vi "array -- find monotonic segments.vi"(6 "min length of monotonic segment":i32=5, 11 "list of numbers":dbl[](array[numeric])=[1.0, 2.0, 3.0, 4.0, 4.0, 5.0, 4.0, 5.0, 3.0, 2.0, 1.0, 1.0, 2.0, 3.0, 4.0, 5.0]) -> (2 "array of monotonic segments":T1[](array[typedef]))   [LabVIEW 2015]
uses:
  array -- monotnic segment.ctl
panel:
  in  "Cluster":T1
  out "ind":i32[](array[numeric])=[1, 2, 3, 4, 4, 5, 4, 5, 3, 2, 1, 1, 2, 3, 4, 5]
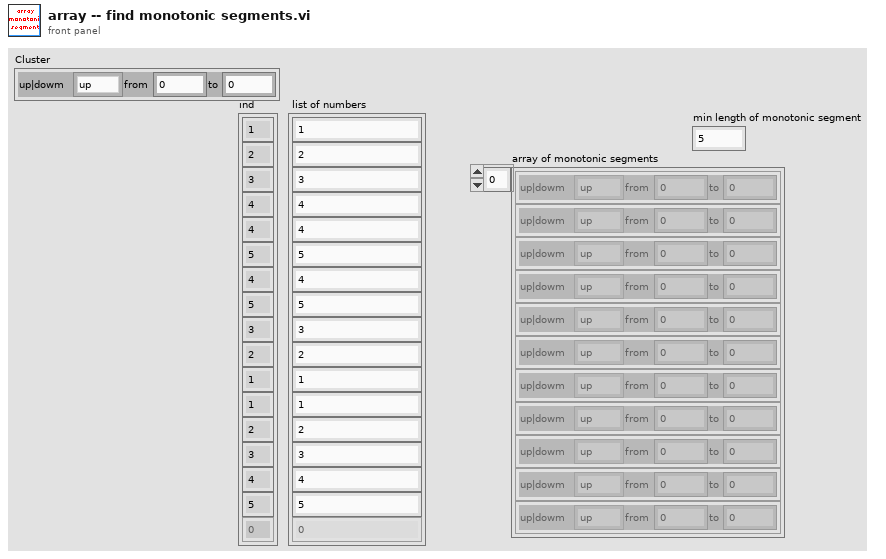
[diagram p1: front panel]
types:
  T1 = typedef "array -- monotnic segment.ctl" = cluster{"to":i32, "from":i32, "up|dowm":enum16{"up", "down"}}
  T2 = cluster{"index to":i32, "index from":i32, "up|dowm":enum16{"up", "down"}}
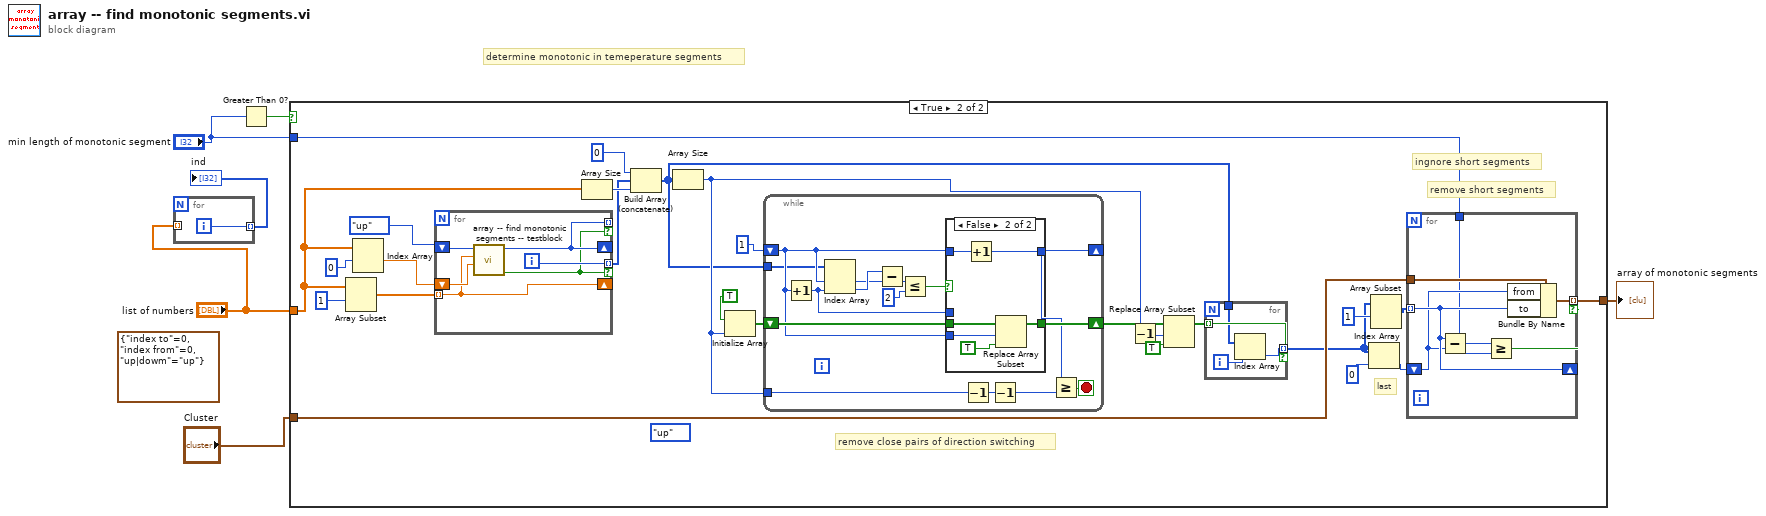
[diagram p0: block diagram]
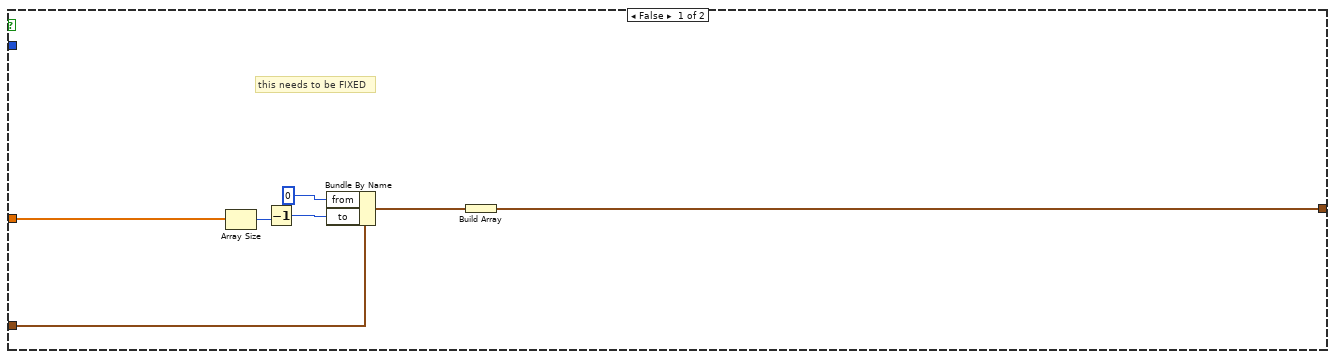
[diagram p2: hidden frame]
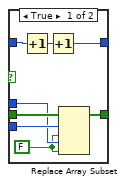
[diagram p3: hidden frame]
diagram:
  (unwired) T2 {"index to"=0, "index from"=0, "up|dowm"=enum."up"}
  # "determine monotonic in temeperature segments"
  n1 = for {
    tunnel: "list of numbers" -> [_] mode=indexing
    tunnel: [w7] -> w4 mode=indexing
    i -> [w7]
  }
  "ind" <- w4
  n2 = Greater Than 0?(x="min length of monotonic segment") -> (x > 0?=w5:bool)
  n3 = case shown="True" w5 {
    tunnel: "list of numbers" -> [w13 w28]
    tunnel: "min length of monotonic segment" -> [_ w15]
    tunnel: "Cluster" -> [w9 w33]
    tunnel: [w8 w18] -> w1
    frame False {
      # "this needs to be FIXED"
      n4 = Array Size(array=w13) -> (size(s)=w12:i32)
      n5 = Decrement(x=w12) -> (x-1=w10:i32)
      n6 = Bundle By Name(cluster=w9, "from"=0 ("index  from"), "to"=w10) -> (w14:T1)
      n7 = Build Array(w14) -> (w8:T1[])
    }
    frame True {
      (unwired) enum16{"up", "down"}."up" ("up|dowm IN")
      # "remove short segments"
      # "last"
      # "remove close pairs of direction switching"
      # "ingnore short segments"
      n8 = Array Subset(array=w28, index=1 ("dimension size")) -> (w38:dbl[])  [unwired: 1 in]
      n9 = Index Array(array=w28, index #1=0 ("dimension size")) -> (element #1=w29:dbl)  [unwired: 1 in, 1 out]
      n10 = for {
        shift-right: [w77] -> _
        shift-left: w29 -> [w78]
        tunnel: w38 -> [w77] mode=indexing
        shift-right: [w75] -> _
        shift-left: enum16{"up", "down"}."up" ("up|dowm IN") -> [w79]
        tunnel: [w76] -> w31 mode=indexing if=w74
        tunnel: [w75] -> _ mode=indexing if=w74
        i -> [w76]
        n11 = call "array -- find monotonic segments -- testblock.vi"("prev"=w78, "next"=w77, "up|dowm IN"=w79) -> ("dir change"=w74:bool, "up|dowm OUT"=w75:enum16{"up", "down"})  [unwired: 7 in]
      }
      n12 = Array Size(array=w28) -> (size(s)=w34:i32)
      n13 = Build Array (concatenate)(0 ("dimension size"), w31, w34) -> (w17:i32[])
      n14 = Array Size(array=w17) -> (size(s)=w23:i32)
      n15 = Initialize Array(TRUE, w23) -> (w26:bool[])
      n16 = while {
        shift-right: [w52] -> w20
        shift-left: w26 -> [w53]
        shift-right: [w41] -> _
        shift-left: 1 ("y") -> [w47]
        tunnel: w23 -> [w46]
        tunnel: w17 -> [w42]
        stop <- w43 stop-if-true
        n17 = Increment(x=w47) -> (x+1=w48:i32)
        n18 = Index Array(array=w42, index #1=w47, index #2=w48) -> (element #1=w50:i32, element #2=w51:i32)
        n19 = Subtract(x=w51, y=w50) -> (x-y=w55:i32)
        n20 = Less Or Equal?(x=w55, y=2) -> (x <= y?=w49:bool)
        n21 = case shown="False" w49 {
          tunnel: w53 -> [w63 w69]
          tunnel: [w62 w68] -> w52
          tunnel: w47 -> [w61 w67]
          tunnel: w48 -> [w60 _]
          tunnel: w47 -> [w58 w65]
          tunnel: [w56 w64] -> w41
          frame True {
            w59 = FALSE
            n22 = Increment(x=w58) -> (x+1=w57:i32)
            n23 = Increment(x=w57) -> (x+1=w56:i32)
            n24 = Replace Array Subset(array=w63, new element #1=w59, index #1=w61, new element #2=w59, index #2=w60) -> (w62:bool[])
          }
          frame False {
            n25 = Increment(x=w65) -> (x+1=w64:i32)
            n26 = Replace Array Subset(array=w69, new element=TRUE, index=w67) -> (w68:bool[])
          }
        }
        n27 = Decrement(x=w46) -> (x-1=w45:i32)
        n28 = Decrement(x=w45) -> (x-1=w44:i32)
        n29 = Greater Or Equal?(x=w41, y=w44) -> (x >= y?=w43:bool)
      }
      n30 = Decrement(x=w23) -> (x-1=w22:i32)
      n31 = Replace Array Subset(array=w20, new element=TRUE, index=w22) -> (w19:bool[])
      n32 = for {
        tunnel: w19 -> [w72] mode=indexing
        tunnel: [w71] -> w16 mode=indexing if=w72
        tunnel: w17 -> [w70]
        i -> [w73]
        n33 = Index Array(array=w70, index=w73) -> (element=w71:i32)
      }
      n34 = Index Array(array=w16, index=0 ("dimension size")) -> (element=w27:i32)
      n35 = Array Subset(array=w16, index=1 ("dimension size")) -> (w35:i32[])  [unwired: 1 in]
      n36 = for {
        tunnel: w33 -> [w86]
        tunnel: w35 -> [w84] mode=indexing
        tunnel: [w85] -> w18 mode=indexing if=w80
        shift-right: [w84] -> _
        shift-left: w27 -> [w83]
        tunnel: w15 -> [w81]
        n37 = Subtract(x=w84, y=w83) -> (x-y=w82:i32)
        n38 = Greater Or Equal?(x=w82, y=w81) -> (x >= y?=w80:bool)
        n39 = Bundle By Name(cluster=w86, "from"=w83, "to"=w84) -> (w85:T1)
      }
    }
  }
  "array of monotonic segments" <- w1
